vi "Position From Buttons.vi"(10 "Current Position":i32, 11 "Buttons":bool[](array[boolean])) -> (3 "Desired Position":i32)   [LabVIEW 2017]
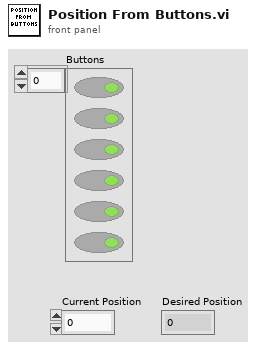
[diagram p1: front panel]
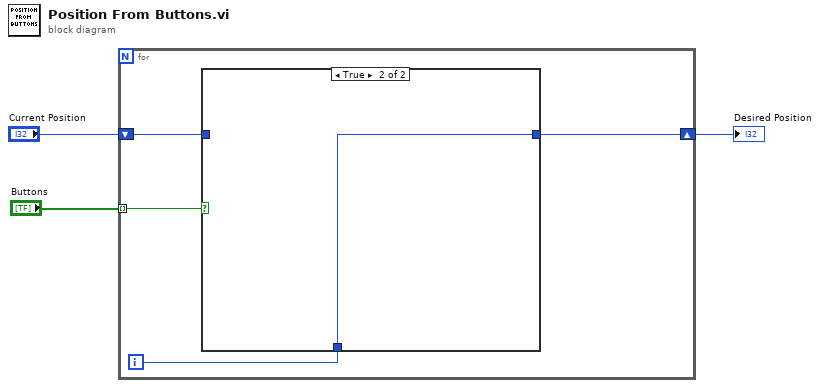
[diagram p0: block diagram]
diagram:
  n1 = for {
    tunnel: "Buttons" -> [w7] mode=indexing
    shift-right: [w4] -> w1
    shift-left: "Current Position" -> [w5]
    i -> [w6]
    n2 = case shown="True" w7 {
      tunnel: [w8 w9] -> w4
      tunnel: w6 -> [_ w9]
      tunnel: w5 -> [w8 _]
      frame False {
      }
      frame True {
      }
    }
  }
  "Desired Position" <- w1
